vi "Global.vi"() -> ()   [LabVIEW 2018]
panel:
  out "Hi_pot_Test(IR)":string[](array[string])
  out "Hi_pot_Test(AC)":string[](array[string])
  out "Product Number":string
  out "MES":dbl
  out "SNLength":dbl
  out "EnabledBarcode":dbl
  out "OperatorNumber":string
  out "WorkOrderNumber":string
  out "TestItemFileNamePath":path
  out "XML文件路径":path[](array[path])
  out "TestFixtureNumber":string
  out "DateTime":string
  out "StatusCode":string
  out "DateTimeEnd":string
  out "DateTimeStart":string
  out "SerialNumber":string
  out "Timestamp":string
  out "EXCLE path":path
  out "TestSN":string
  in  "RS232_6":refnum<visa-resource-name>
  out "GetDriverFileName":string
  out "GetDriverFilePath":path
  in  "GPIB_5":refnum<visa-resource-name>
  in  "GPIB_4":refnum<visa-resource-name>
  in  "GPIB_3":refnum<visa-resource-name>
  in  "GPIB_2":refnum<visa-resource-name>
  in  "GPIB_1":refnum<visa-resource-name>
  in  "PCICard5":refnum<visa-resource-name>
  in  "PCICard4":refnum<visa-resource-name>
  in  "PCICard3":refnum<visa-resource-name>
  in  "PCICard2":refnum<visa-resource-name>
  in  "PCICard1":refnum<visa-resource-name>
  in  "RS232_5":refnum<visa-resource-name>
  in  "RS232_4":refnum<visa-resource-name>
  in  "RS232_3":refnum<visa-resource-name>
  in  "RS232_2":refnum<visa-resource-name>
  in  "RS232_1":refnum<visa-resource-name>
  in  "USB5":refnum<visa-resource-name>
  in  "USB4":refnum<visa-resource-name>
  in  "USB3":refnum<visa-resource-name>
  in  "USB":refnum<visa-resource-name> caption="USB2"
  in  "USB1":refnum<visa-resource-name>
  out "MainPath":path
  out "GUI":path
  out "max_symbols":path
  out "Edit":bool
  out "Save Database path":path
  out "XLM path":path
  out "TXT path":path
  out "CSV path":path
  out "Test_Message":T1
  out "Test Setup":i32=12
  out "Barcode Length":i32=12
  out "HW Config File":path
  out "SaveProgramFile":string
  out "ConfigPath":path
  out "ModelInformation":path
  out "LogPath":path
  # "测试项目驱动"
  # "fixture_Driver"
  # "Hi-pot_Driver"
  # "2020-07-17T14:35:07"
  # "KC3404KB700731"
  # "2020-07-17T14:35:11"
  # "2020-07-17T14:35:07"
  # "PASS/FAIL"
  # "2020-07-14T13:13:44"
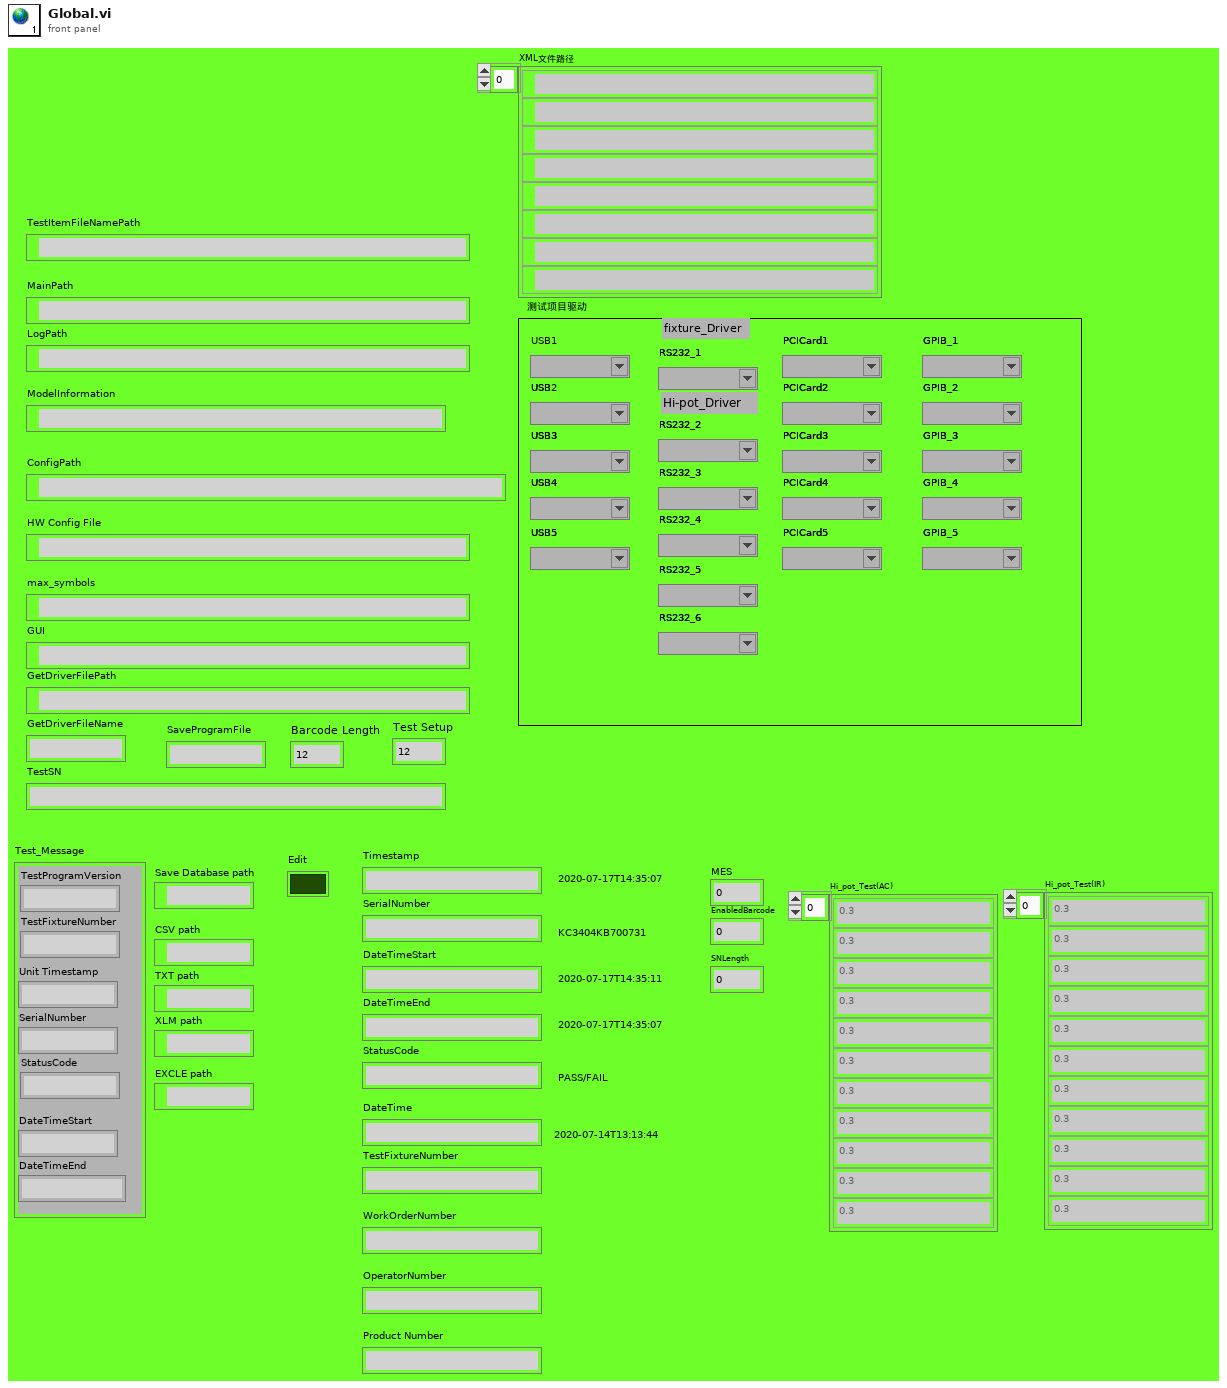
[diagram p1: front panel]
types:
  T1 = cluster{"Unit Timestamp":string, "SerialNumber":string, "StatusCode":string, "DateTimeStart":string, "DateTimeEnd":string, "TestProgramVersion":string, "TestFixtureNumber":string}
diagram:
